vi "SysTest-Is Cal Mic Selected.vi"(10 "input selections":i32[](array[numeric]), 11 "AI Names":string[](array[string])) -> (1 "Cal mic index":i32, 3 "Cal mic selected?":bool)   [LabVIEW 2020]
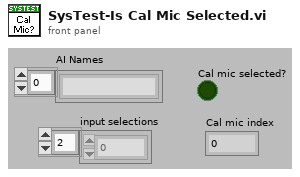
[diagram p1: front panel]
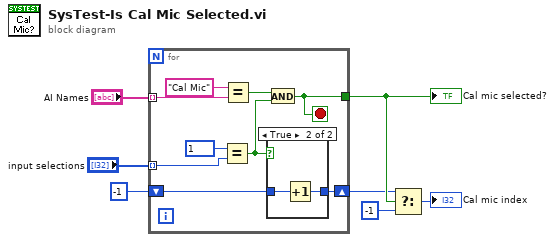
[diagram p0: block diagram]
diagram:
  n1 = for {
    tunnel: "AI Names" -> [w16] mode=indexing
    tunnel: "input selections" -> [w11] mode=indexing
    tunnel: [w12] -> w5
    shift-right: [w8] -> w1
    shift-left: -1 -> [w9]
    stop <- w12 stop-if-true
    n2 = Equal?(x=1, y=w11) -> (x = y?=w10:bool)
    n3 = Equal?(x="Cal Mic", y=w16) -> (x = y?=w13:bool)
    n4 = case shown="True" w10 {
      tunnel: w9 -> [w17 w19]
      tunnel: [w17 w18] -> w8
      frame False {
      }
      frame True {
        n5 = Increment(x=w19) -> (x+1=w18:i32)
      }
    }
    n6 = And(x=w13, y=w10) -> (x .and. y?=w12:bool)
  }
  "Cal mic selected?" <- w5
  n7 = Select(t=w1, s=w5, f=-1) -> (s? t:f=→"Cal mic index":i32)
